vi "624FPGA_SystemStart Async Agent.vi"(8 "error in":errorcluster) -> (0 "error out":errorcluster)   [LabVIEW 2013]
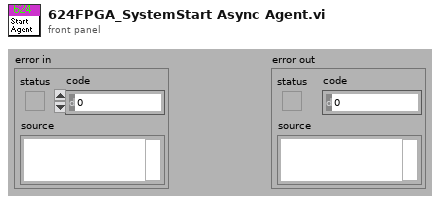
[diagram p1: front panel]
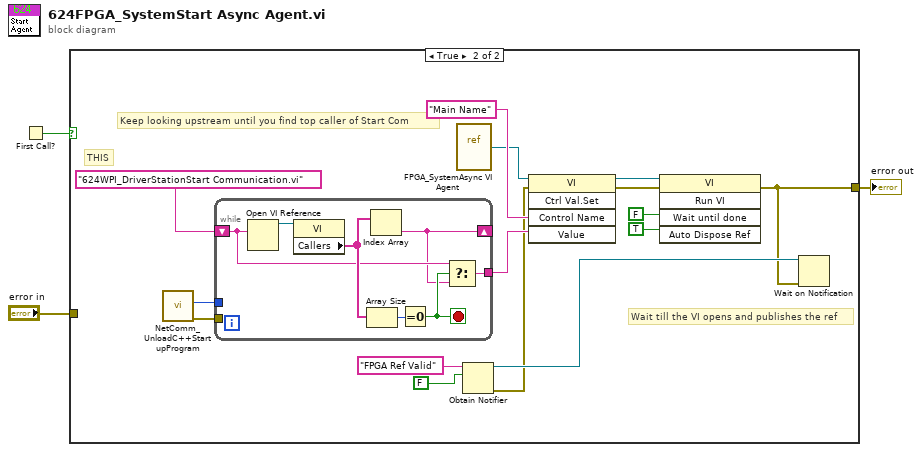
[diagram p0: block diagram]
diagram:
  n1 = First Call?() -> (First Call?: T/F=w3:bool)
  n2 = case shown="True" w3 {
    tunnel: [w4 w10] -> w2
    tunnel: "error in" -> [w4 _]
    frame False {
    }
    frame True {
      # "THIS"
      # "Wait till the VI opens and publishes the ref"
      # "Keep looking upstream until you find top caller of Start Com"
      n3 = call <vilib>:"NetComm_UnloadC++StartupProgram.vi"() -> ("error out"=w6:errorcluster, "return code"=w5:i32)  [unwired: 1 in, 9 out]
      n4 = while {
        shift-right: [w21] -> _
        shift-left: "624WPI_DriverStationStart Communication.vi" -> [w22]
        tunnel: [w20] -> w13
        tunnel: w6 -> [_]
        tunnel: w5 -> [_]
        stop <- w23 stop-if-true
        n5 = Open VI Reference(vi path=w22) -> (vi reference=w26:refnum<vi>)  [unwired: 1 in, 5 out]
        n6 = property class="VI"(reference=w26) -> ("Callers"=w24:string[])  [unwired: 1 in, 2 out]
        n7 = Array Size(array=w24) -> (size(s)=w25:i32)
        n8 = Index Array(array=w24) -> (element=w21:string)  [unwired: 1 in]
        n9 = Equal To 0?(x=w25) -> (x = 0?=w23:bool)
        n10 = Select(t=w22, s=w23, f=w21) -> (s? t:f=w20:string)
      }
      n11 = vi-ref <vilib>:"FPGA_SystemAsync VI Agent.vi"() -> (w15:refnum<vi>)
      n12 = Obtain Notifier(name (unnamed)="FPGA Ref Valid", notification data type=FALSE) -> (notifier out=w11:refnum<notifier>, error out=w7:errorcluster)  [unwired: 2 in, 1 out]
      n13 = invoke class="VI" method="Ctrl Val.Set"(reference=w15, error in=w7, "Control Name"="Main Name", "Value"=w13) -> (reference out=w17:refnum<vi>, error out=w14:errorcluster)  [unwired: 1 in, 3 out]
      n14 = invoke class="VI" method="Run VI"(reference=w17, error in=w14, "Wait until done"=FALSE ("Wait Until Done"), "Auto Dispose Ref"=TRUE ("Auto Dispose Reference")) -> (error out=w10:errorcluster)  [unwired: 1 in, 4 out]
      n15 = Wait on Notification(notifier=w11, error in (no error)=w10) -> ()  [unwired: 6 out]
    }
  }
  "error out" <- w2
